vi "close.vi"(8 "error in (no error)":errorcluster, 11 "Table in":refnum<class "Table.lvclass">) -> (0 "error out":errorcluster)   [LabVIEW 2020, in "toml_edit.lvlib" / "Table.lvclass"]
uses:
  Table.lvclass
  Table.lvclass/Table.ctl
  dragon_toml_64.dll
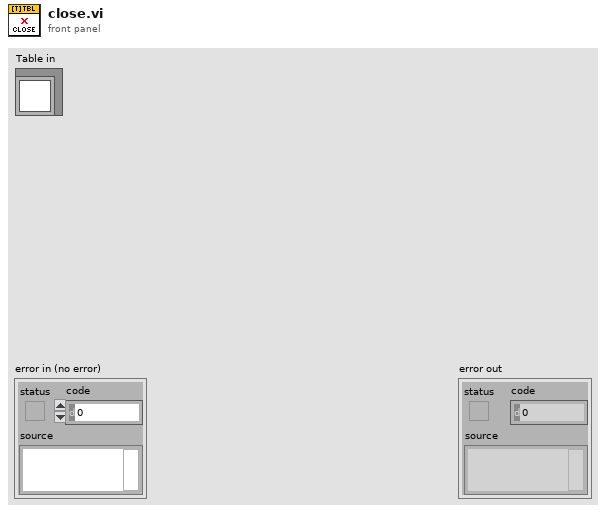
[diagram p1: front panel]
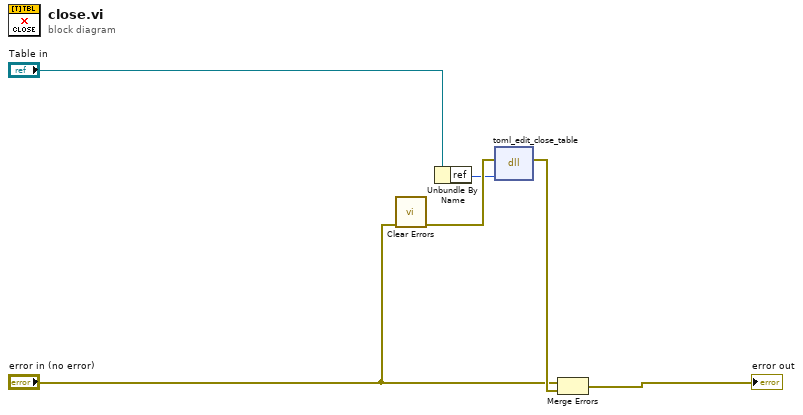
[diagram p0: block diagram]
diagram:
  n1 = call <vilib>:"Clear Errors.vi"("error in (no error)"="error in (no error)") -> ("error out"=w5:errorcluster)  [unwired: 5 in, 1 out]
  n2 = Unbundle By Name("Table in") -> ("ref"=w4:u64)
  n3 = dll-call lib="C:/Projects/toml-edit-labview/lv_src/dragon_toml_*.dll" fn="toml_edit_close_table"(error in=w5, "ptr"=w4) -> (error out=w6:errorcluster)  [unwired: 4 in, 1 out]
  n4 = Merge Errors("error in (no error)", w6) -> (→"error out":errorcluster)
